vi "AutoDrive.vi"() -> ()   [LabVIEW 2013]
uses:
  <vilib>/addons/control/pid/pid.llb/PID (DBL).vi
  <vilib>/Rock Robotics/WPI/RobotDrive/WPI_RobotDriveGetSetRefNum.vi
  <vilib>/addons/control/pid/NI_PID_pid.lvlib
panel:
  in  "Input":dbl format="%#_13g"
  in  "D 2":dbl
  in  "I 2":dbl=0.01
  in  "P 2":dbl=1.0
  out "Encoder Distance":cluster{"Rate":dbl, "Rate":dbl}
  out "error out 2":errorcluster
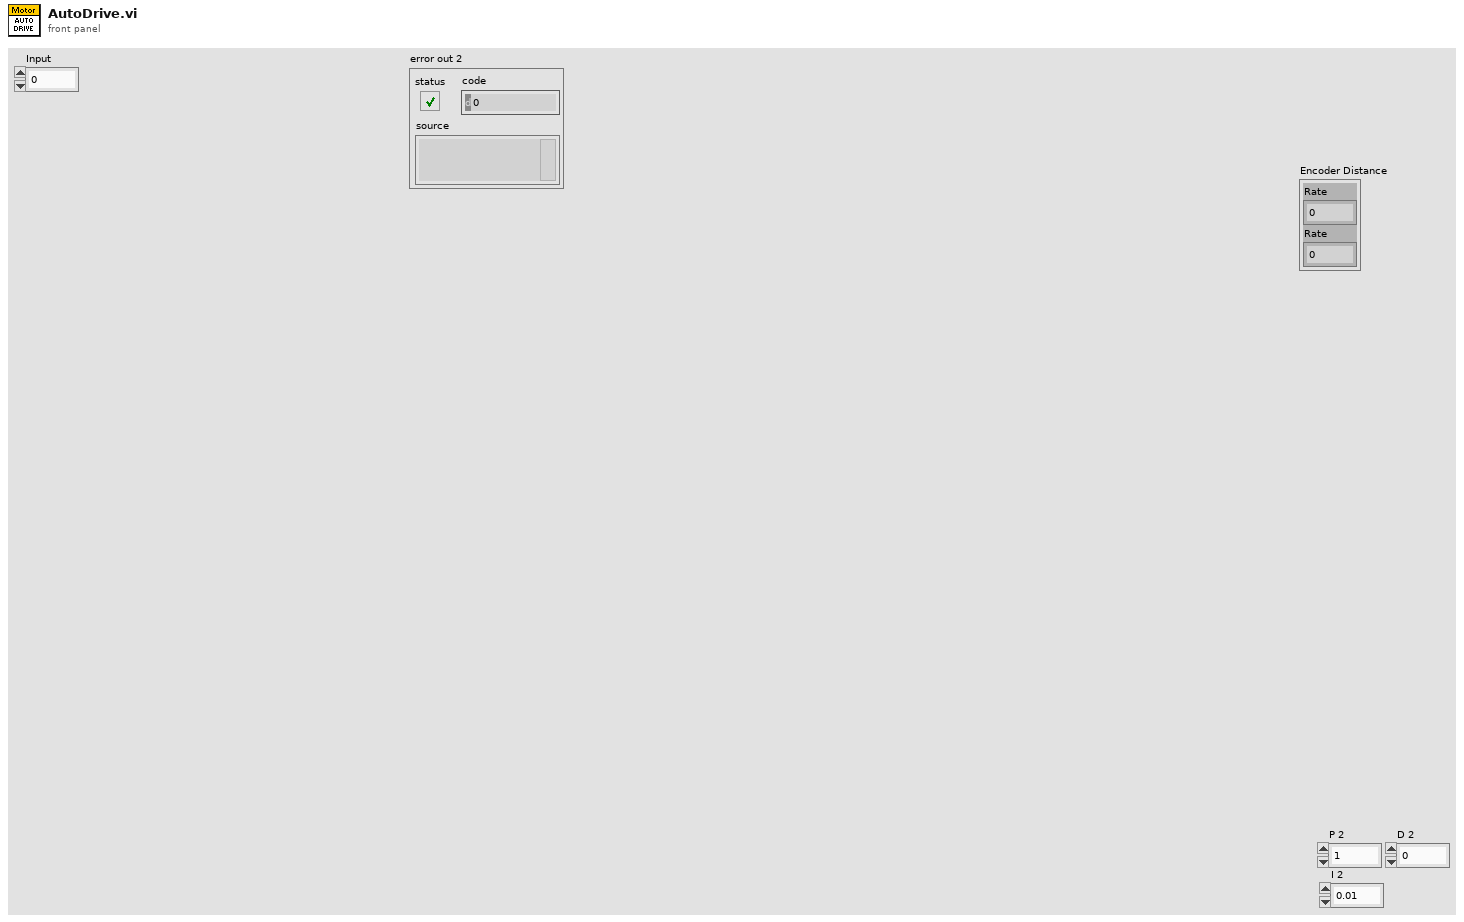
[diagram p1: front panel]
types:
  T1 = typedef "WPI_RobotDriveDevRef.ctl" = cluster{"DevStatus":errorcluster, "Motors[]":T2[], "Square Inputs":bool, "Max Output":dbl, "Isochronous":bool}
  T2 = typedef "WPI_MotorControlDeviceRef.ctl" = cluster{"DeviceStatus":errorcluster, "Type":enum16{"PWM", "CAN"}, "PWM":cluster{"Digital Module":T3, "PWM Channel":T4, "DeadBand":T5}, "CAN":cluster{"Device Number":u8, "Control Mode":T6, "Semaphore":T7, "Max Vout":dbl}, "Invert":bool, "TransformRef":T8, "InvTransformRef":T8}
  T3 = typedef "FPGA_TypedefDigitalModule.ctl" = enum16{"Digital Module 1", "Digital Module 2"}
  T4 = typedef "FPGA_DIOPWMChannel.ctl" = enum8{"PWM 1", "PWM 2", "PWM 3", "PWM 4", "PWM 5", "PWM 6", "PWM 7", "PWM 8", "PWM 9", "PWM 10", "Invalid"}
  T5 = typedef "WPI_PWMDeadband.ctl" = cluster{"Name":string, "maxPositivePwm":i32, "minPositivePwm":i32, "centerPwm":i32, "maxNegativePwm":i32, "minNegativePwm":i32, "angularRange":u16}
  T6 = typedef "WPI_CANJaguar_ControlMode.ctl" = enum8{"Percent VBus", "Current", "Speed", "Position", "Voltage"}
  T7 = typedef "Semaphore RefNum" = refnum<k1>
  T8 = typedef "WPI_PWMTransform_ConPane.ctl" = refnum<vi>
  T9 = typedef "WPI_EncoderDevRef.ctl" = cluster{"DevStatus":errorcluster, "EncoderIndex":T10, "CounterIndex":T11, "DistancePerCount":dbl, "Decoding Type":T12}
  T10 = typedef "FPGA_EncoderIdx.ctl" = enum8{"Enc 0", "Enc 1", "Enc 2", "Enc 3", "Invalid"}
  T11 = typedef "FPGA_CounterCtrSystemIndex.ctl" = enum8{"Ctr 0", "Ctr 1", "Ctr 2", "Ctr 3", "Ctr 4", "Ctr 5", "Ctr 6", "Ctr 7", "Invalid"}
  T12 = typedef "WPI_EncoderType.ctl" = enum16{"1x", "2x", "4x"}
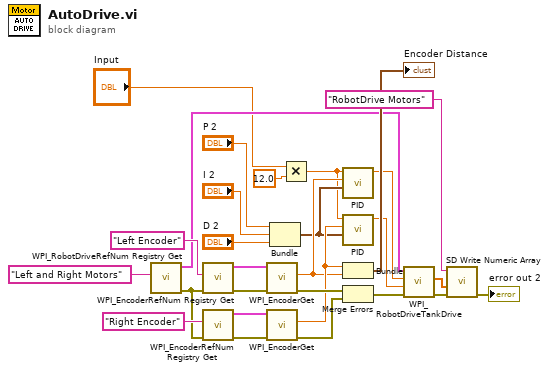
[diagram p0: block diagram]
diagram:
  n1 = call <vilib>:"WPI_RobotDriveRefNum Registry Get.vi"("refnum name"="Left and Right Motors") -> ("error out"=w9:errorcluster, "RobotDriveDevRef"=w8:T1)  [unwired: 9 in]
  n2 = call <vilib>:"WPI_EncoderRefNum Registry Get.vi"("error in (no error)"=w9, "refnum name"="Left Encoder") -> ("error out"=w27:errorcluster, "EncoderDevRef"=w26:T9)  [unwired: 8 in]
  n3 = call <vilib>:"WPI_EncoderRefNum Registry Get.vi"("error in (no error)"=w9, "refnum name"="Right Encoder") -> ("error out"=w25:errorcluster, "EncoderDevRef"=w24:T9)  [unwired: 8 in]
  n4 = call <vilib>:"WPI_EncoderGet.vi"("error in (no error)"=w27, "EncoderDevRef"=w26) -> ("error out"=w22:errorcluster, "Distance"=w14:dbl)  [unwired: 4 in, 4 out]
  n5 = call <vilib>:"WPI_EncoderGet.vi"("error in (no error)"=w25, "EncoderDevRef"=w24) -> ("error out"=w21:errorcluster, "Distance"=w15:dbl)  [unwired: 4 in, 4 out]
  n6 = Bundle("P 2"="P 2", "I 2"="I 2", "D 2"="D 2") -> (w10:cluster{"P 2":dbl, "I 2":dbl, "D 2":dbl})  [unwired: 1 in]
  n7 = Multiply(x="Input", y=12.0) -> (x*y=w1:dbl)
  n8 = call-poly <vilib>:"PID.vi"("PID gains"=w10, "process variable"=w14, "setpoint"=w1) -> ("output"=w4:dbl)  [unwired: 7 in, 1 out]
  n9 = call-poly <vilib>:"PID.vi"("PID gains"=w10, "process variable"=w15, "setpoint"=w1) -> ("output"=w5:dbl)  [unwired: 7 in, 1 out]
  n10 = Bundle("Distance"=w15, "Distance"=w14) -> (→"Encoder Distance":cluster{"Distance":dbl, "Distance":dbl})  [unwired: 1 in]
  n11 = Merge Errors(w22, w21) -> (w20:errorcluster)
  n12 = call <vilib>:"WPI_RobotDriveTankDrive.vi"("error in (no error)"=w20, "Right axis value"=w5, "Left axis value"=w4, "RobotDriveDevRef"=w8) -> ("error out"=w19:errorcluster, "Motor Values"=w18:dbl[])  [unwired: 5 in, 1 out]
  n13 = call <vilib>:"SD Write Numeric Array.vi"("error in"=w19, "Numeric Array"=w18, "Name"="RobotDrive Motors") -> ("error out"=→"error out 2":errorcluster)  [unwired: 7 in, 1 out]
